vi "DecodeMonitorHeader(BECW).vi"(11 "becw":u32=5322999 format="%.0b") -> (3 "BECW":T1)   [LabVIEW 2020, in "AIM664LV.lvlib"]
uses:
  AIM664LV.lvlib
  _controls/monitor_becw_type.ctl
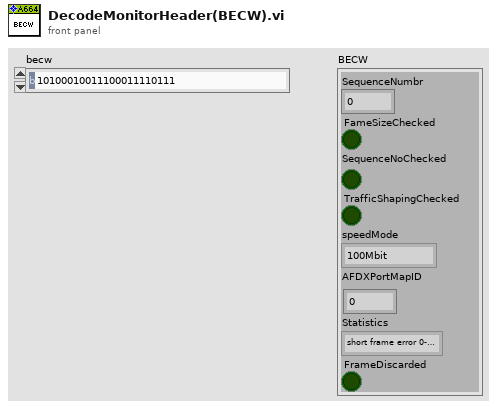
[diagram p1: front panel]
types:
  T1 = typedef "AIM664LV.lvlib/monitor_becw_type.ctl" = cluster{"SequenceNumbr":u8, "FameSizeChecked":bool, "SequenceNoChecked":bool, "TrafficShapingChecked":bool, "speedMode":enum16{"100Mbit", "10Mbit", "1Gbit"}, "AFDXPortMapID":u8, "Statistics":enum16{"short frame error 0-63Bytes", "64-127 Bytes", "128-255 Bytes", "256-511 Bytes", "512-1023 Bytes", "1024-1518 Bytes", ">1518 Bytes"}, "FrameDiscarded":bool}
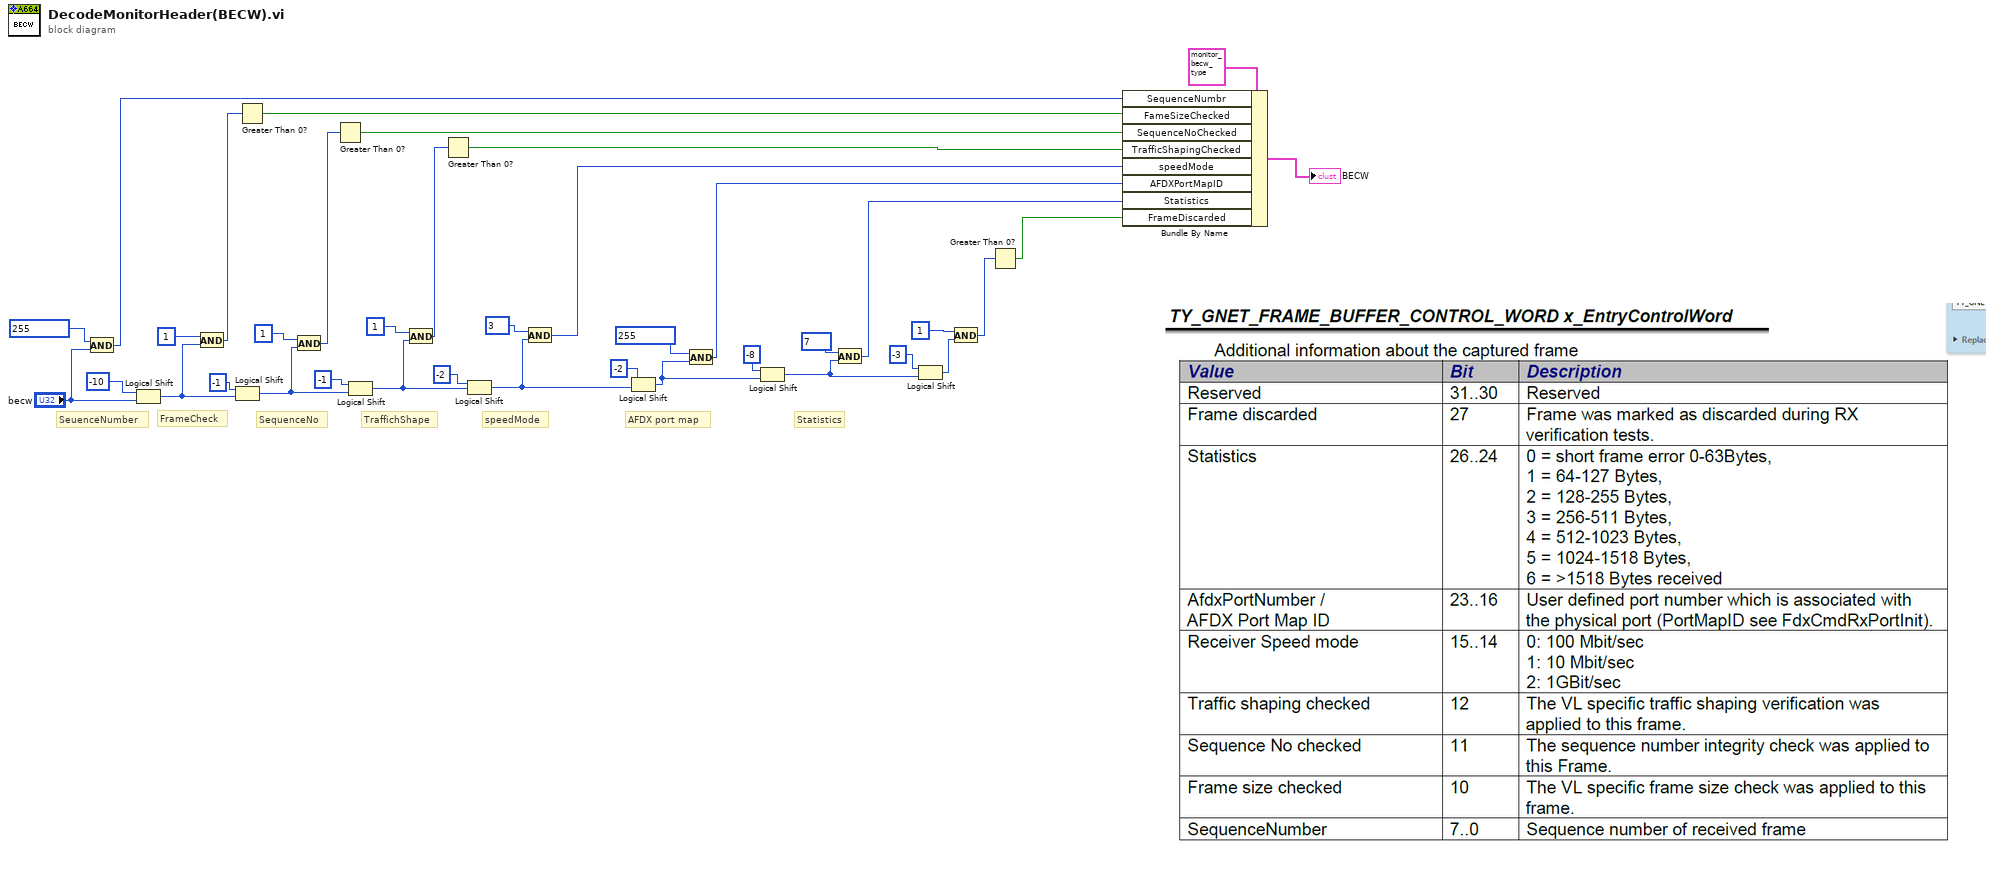
[diagram p0: block diagram]
diagram:
  # "Statistics"
  # "AFDX port map"
  # "speedMode"
  # "TraffichShape"
  # "SequenceNo"
  # "FrameCheck"
  # "SeuenceNumber"
  n1 = And(x=u32 255 ("Numeric"), y="becw") -> (x .and. y?=w4:u32)
  n2 = Logical Shift(y=i16 -10, x="becw") -> (x << y=w24:u32)
  n3 = And(x=u32 1 ("Numeric"), y=w24) -> (x .and. y?=w26:u32)
  n4 = Logical Shift(y=i16 -1, x=w24) -> (x << y=w19:u32)
  n5 = Greater Than 0?(x=w26) -> (x > 0?=w25:bool)
  n6 = And(x=u32 1 ("Numeric"), y=w19) -> (x .and. y?=w21:u32)
  n7 = Greater Than 0?(x=w21) -> (x > 0?=w20:bool)
  n8 = Logical Shift(y=i16 -1, x=w19) -> (x << y=w12:u32)
  n9 = And(x=u32 1 ("Numeric"), y=w12) -> (x .and. y?=w16:u32)
  n10 = Greater Than 0?(x=w16) -> (x > 0?=w15:bool)
  n11 = Logical Shift(y=i16 -2, x=w12) -> (x << y=w9:u32)
  n12 = And(x=u32 3 ("Numeric"), y=w9) -> (x .and. y?=w10:u32)
  n13 = Logical Shift(y=i16 -2, x=w9) -> (x << y=w7:u32)
  n14 = And(x=u32 255 ("Numeric"), y=w7) -> (x .and. y?=w8:u32)
  n15 = Logical Shift(y=i16 -8, x=w7) -> (x << y=w33:u32)
  n16 = And(x=u32 7 ("Numeric"), y=w33) -> (x .and. y?=w2:u32)
  n17 = Logical Shift(y=i16 -3, x=w33) -> (x << y=w28:u32)
  n18 = And(x=u32 1 ("Numeric"), y=w28) -> (x .and. y?=w3:u32)
  n19 = Greater Than 0?(x=w3) -> (x > 0?=w1:bool)
  n20 = Bundle By Name(cluster=T1 {"SequenceNumbr"=0, "FameSizeChecked"=FALSE, "SequenceNoChecked"=FALSE, "TrafficShapingChecked"=FALSE, "speedMode"=enum."100Mbit", "AFDXPortMapID"=0, "Statistics"=enum."short frame error 0-63Bytes", "FrameDiscarded"=FALSE}, "SequenceNumbr"=w4, "FameSizeChecked"=w25, "SequenceNoChecked"=w20, "TrafficShapingChecked"=w15, "speedMode"=w10, "AFDXPortMapID"=w8, "Statistics"=w2, "FrameDiscarded"=w1) -> (→"BECW":T1)
